vi "lm Assign LE Colors.vi"(8 "error in (no error)":errorcluster, 11 "strColorArray":string) -> (0 "error out":errorcluster, 2 "function return":i32, 3 "strColorArray out":string)   [LabVIEW 2017, in "LumencorDLLDbg64.lvlib"]
doc: "This function is used to also assign\\Modeify Colors in the LE Color map. It does not change the color display but rather the color channel associated with each color. Only use this function if instructed to by Lumencor.\n\n\n\n\nextern \"C\" LUMENCORDLL2B_API int lmAssignLEColors(char *strColorArray);"
uses:
  LumencorDLLDbg64.lvlib
  LumencorDLLDbg64.dll
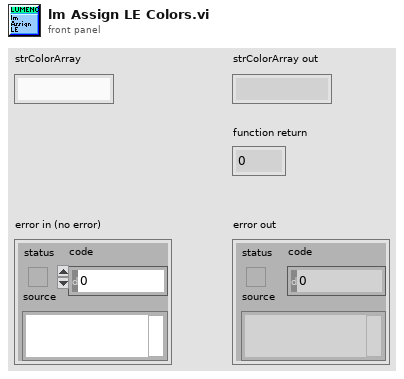
[diagram p1: front panel]
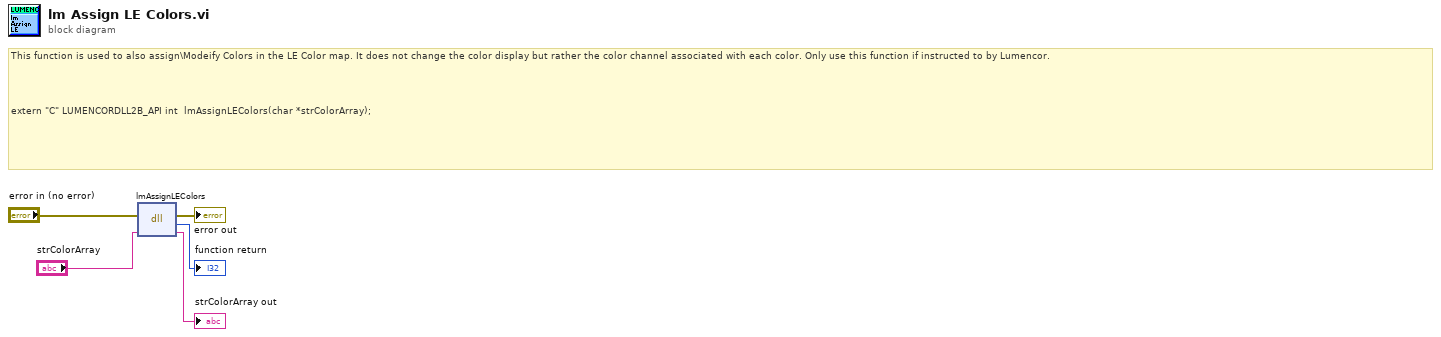
[diagram p0: block diagram]
diagram:
  # "This function is used to also assign\\Modeify Colors in the LE Color map. It does not change the color display but rather the color channel associated with each color. Only use this function if instructed to by Lumencor.\n\n\n\n\nextern \"C\" LUMENCORDLL2B_API int  lmAssignLEColors(char *strColorArray);"
  n1 = dll-call lib="Q:/GIT -- Lumencor DLL4/LabVIEW Library (64bit)/LumencorDLLDbg64.*" fn="lmAssignLEColors"(error in="error in (no error)", "strColorArray"="strColorArray") -> (error out=→"error out":errorcluster, →"function return":i32, "strColorArray"=→"strColorArray out":string)  [unwired: 2 in, 1 out]
